vi "Setup.vi"(8 "error in":errorcluster, 9 "Path":path, 10 "Name":string) -> (0 "error out":errorcluster, 3 "Launcher out":refnum<class "Launcher.lvclass">)   [LabVIEW 2023, in "Launcher.lvlib" / "Launcher.lvclass"]
uses:
  Library/Launcher.lvclass
  Library/Launcher.lvclass/Launcher.ctl
  Accessors/Write Name.vi
  Accessors/Write Path.vi
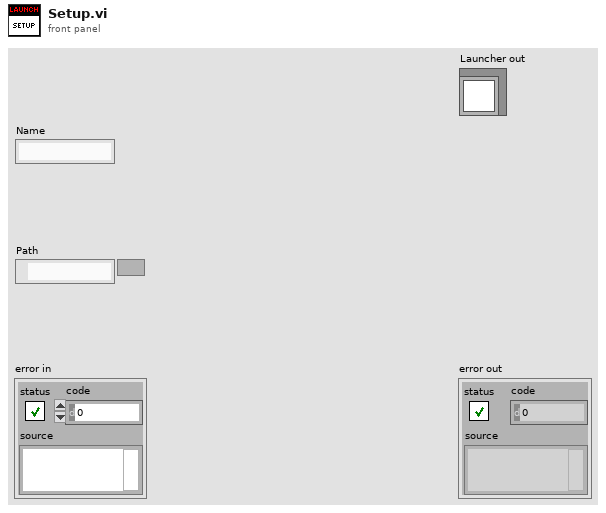
[diagram p1: front panel]
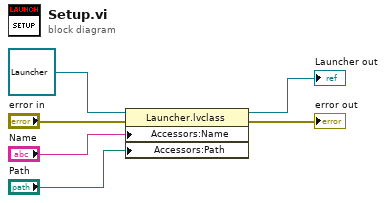
[diagram p0: block diagram]
diagram:
  n1 = property class="Launcher.lvclass"(reference=refnum<class "Launcher.lvclass"> refnum ("Launcher in"), error in="error in", "Accessors:Name"="Name", "Accessors:Path"="Path") -> (reference out=→"Launcher out":refnum<class "Launcher.lvclass">, error out=→"error out":errorcluster)
